vi "Read Ring Refnum.vi"(8 "error in (no error)":errorcluster, 11 "Ring Field in":refnum<class "Ring Field.lvclass">) -> (0 "error out":errorcluster, 2 "Ring Refnum":refnum<vi>, 3 "Ring Field out":refnum<class "Ring Field.lvclass">)   [LabVIEW 2020, in "Ring Field.lvclass"]
uses:
  Ring Field.lvclass
  C:/Users/User/Desktop/Raman Program/Database OOP/source/Field/Field.lvclass
  Field.lvclass/Field.ctl
  Field.lvclass
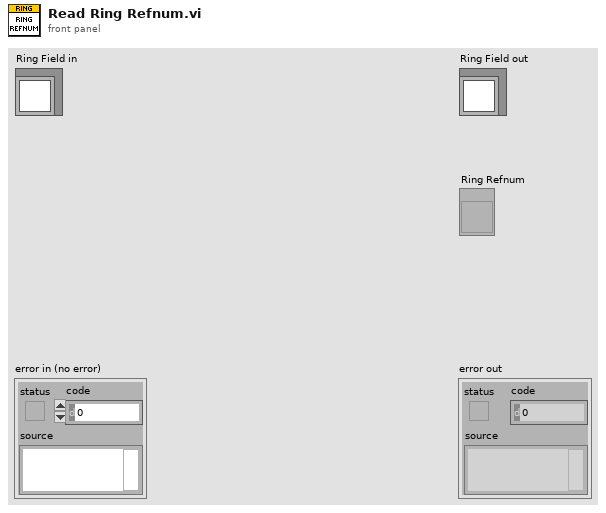
[diagram p1: front panel]
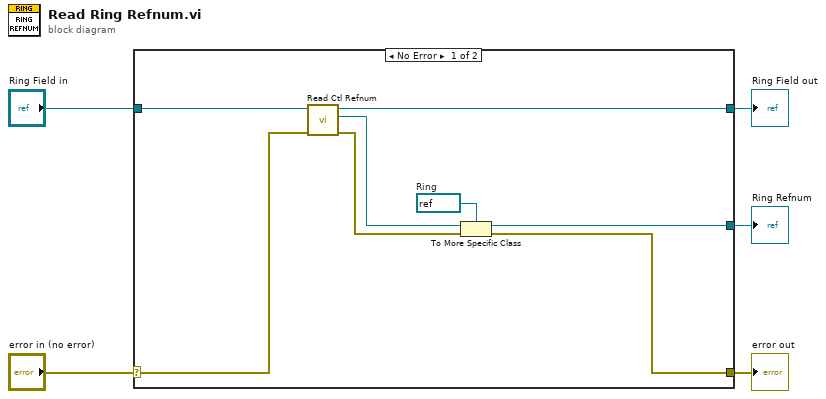
[diagram p0: block diagram]
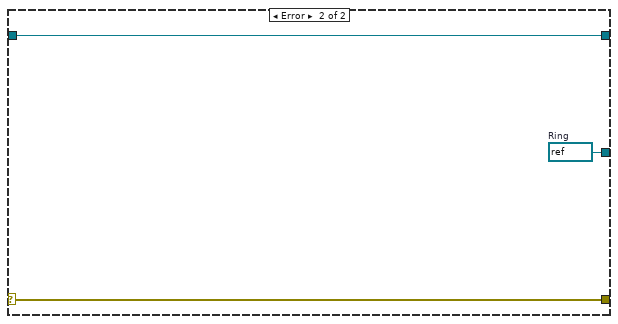
[diagram p2: hidden frame]
diagram:
  n1 = case shown="No Error" "error in (no error)" {
    selector: "error in (no error)" -> [w8 w16]
    tunnel: [w6 w16] -> w4
    tunnel: [w12 w15] -> w2
    tunnel: "Ring Field in" -> [w13 w15]
    tunnel: [w9 w14] -> w1
    frame No Error {
      w10 = refnum<vi> refnum  # Ring
      n2 = call "Read Ctl Refnum.vi"("error in (no error)"=w8, "Field in"=w13) -> ("error out"=w7:errorcluster, "Ctl Refnum"=w11:refnum<vi>, "Field out"=w12:refnum<class "Ring Field.lvclass">)  [unwired: 7 in]
      n3 = To More Specific Class(target class=w10, reference=w11, error in=w7) -> (specific class reference=w9:refnum<vi>, error out=w6:errorcluster)
    }
    frame Error {
      w14 = refnum<vi> refnum  # Ring
    }
  }
  "error out" <- w4
  "Ring Field out" <- w2
  "Ring Refnum" <- w1
